vi "Get Audio Device Volume.vi"(8 "error in (no error)":errorcluster, 11 "Audio Device Refnum In":T1) -> (0 "error out":errorcluster, 2 "Volume":sgl, 3 "Audio Device Refnum Out":T1)   [LabVIEW 2020, in "G-Audio.lvlib"]
doc: "Wait for the audio device to finish playback of all audio data in its buffer.\n\nWill return an error if used with a capture audio device."
uses:
  G-Audio.lvlib
  Controls/Audio Device Refnum.ctl
  <vilib>/Utility/error.llb/Error Cluster From Error Code.vi
  lib/g_audio_32.dll
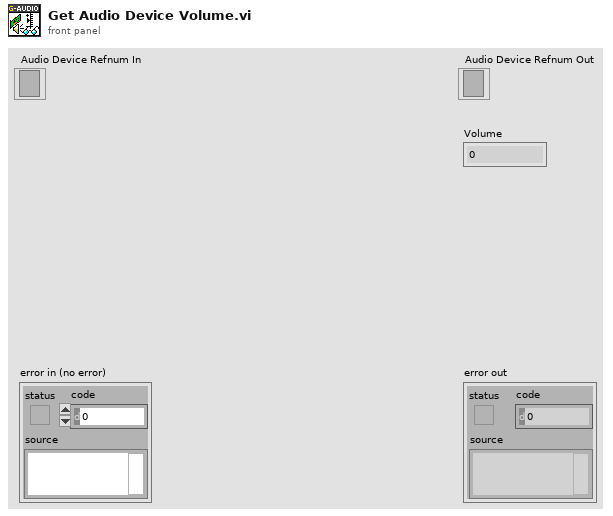
[diagram p1: front panel]
types:
  T1 = typedef "G-Audio.lvlib/Audio Device Refnum.ctl" = refnum<file>
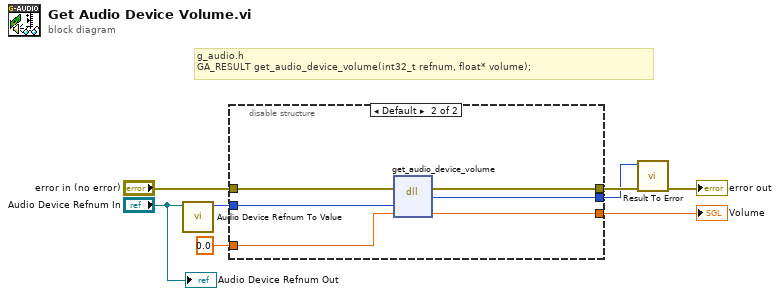
[diagram p0: block diagram]
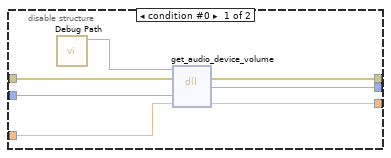
[diagram p2: hidden frame]
diagram:
  # "g_audio.h\nGA_RESULT get_audio_device_volume(int32_t refnum, float* volume);"
  n1 = call "Audio Device Refnum To Value.vi"("Audio Device Refnum"="Audio Device Refnum In") -> ("Refnum Value"=w6:i32)  [unwired: 10 in]
  n2 = disable-structure shown="Default" {
    disable-tunnel: [w14 w21] -> w8
    disable-tunnel: [w13 w20] -> w7
    disable-tunnel: w6 -> [w12 w19]
    disable-tunnel: "error in (no error)" -> [w11 w18]
    disable-tunnel: sgl 0.0 ("volume") -> [w10 w17]
    disable-tunnel: [w9 w16] -> w1
    frame condition #0 {
      n3 = call "Debug Path.vi"() -> ("Debug Path"=w15:path)  [unwired: 11 in]
      n4 = dll-call lib="?" fn="get_audio_device_volume"(path in=w15, error in=w11, "refnum"=w12, "volume"=w10) -> (error out=w14:errorcluster, "result"=w13:i32, "volume"=w9:sgl)  [unwired: 2 in, 1 out]
    }
    frame condition #1 (active) {
      n5 = dll-call lib="C:/github/dataflowg/g-audio/src/LabVIEW/G-Audio/lib/g_audio_*.*" fn="get_audio_device_volume"(error in=w18, "refnum"=w19, "volume"=w17) -> (error out=w21:errorcluster, "result"=w20:i32, "volume"=w16:sgl)  [unwired: 3 in, 1 out]
    }
  }
  "Volume" <- w1
  n6 = call "Result To Error.vi"("error in (no error)"=w8, "Result Code"=w7) -> ("error out"=→"error out":errorcluster)  [unwired: 9 in]
  "Audio Device Refnum Out" <- "Audio Device Refnum In"
